vi "Write tcpSettings.vi"(8 "error in (no error)":errorcluster, 10 "tcpSettings":T1={"IP"="127.0.0.1", "port"=50000, "connection_timeout "=10, "reading_timeout"=10, "writing_timeout"=10}, 11 "TCPClient in":refnum<class "TCPClient.lvclass">) -> (0 "error out":errorcluster, 3 "TCPClient out":refnum<class "TCPClient.lvclass">)   [LabVIEW 2016, in "tcp.lvlib" / "TCPClient.lvclass"]
uses:
  TCPClient.lvclass
  tcpTypedefs/TCPSettings.ctl
  TCPClient.lvclass/TCPClient.ctl
  tcp.lvlib
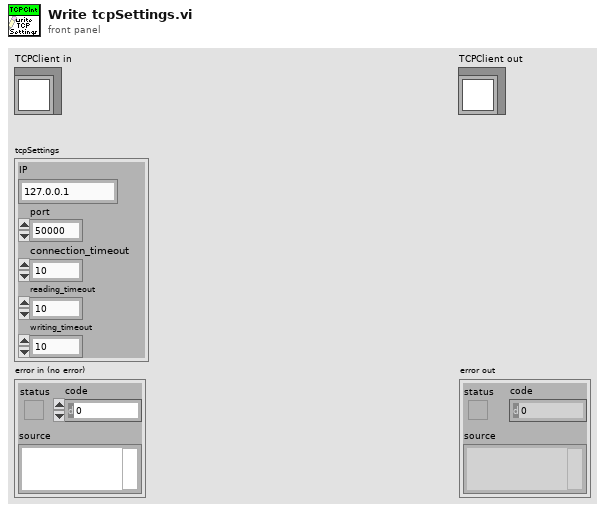
[diagram p1: front panel]
types:
  T1 = typedef "tcp.lvlib/TCPSettings.ctl" = cluster{"IP":string, "port":u16, "connection_timeout ":i32, "reading_timeout":i32, "writing_timeout":i32}
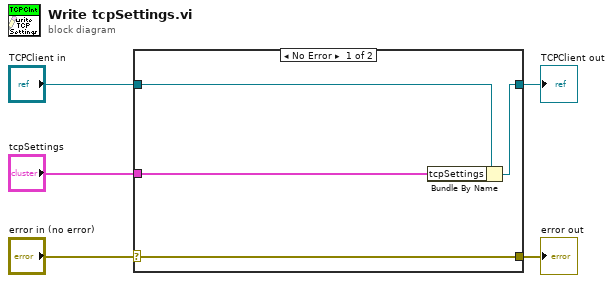
[diagram p0: block diagram]
diagram:
  n1 = case shown="No Error" "error in (no error)" {
    selector: "error in (no error)" -> [w9 w10]
    tunnel: [w9 w10] -> w4
    tunnel: [w7 w11] -> w2
    tunnel: "TCPClient in" -> [w8 w11]
    tunnel: "tcpSettings" -> [w6 _]
    frame No Error {
      n2 = Bundle By Name(cluster=w8, "tcpSettings"=w6) -> (w7:refnum<class "TCPClient.lvclass">)
    }
    frame Error {
    }
  }
  "error out" <- w4
  "TCPClient out" <- w2
